vi "Add Step at Index.vi"(8 "error in (no error)":errorcluster, 9 "Step":refnum<class "Step.lvclass">, 10 "Index":i32, 11 "SequenceViewPanel in":refnum<class "SequenceViewPanel.lvclass">) -> (0 "error out":errorcluster, 1 "Step Group":T1, 2 "Parent Tag":string, 3 "SequenceViewPanel out":refnum<class "SequenceViewPanel.lvclass">)   [LabVIEW 2020, in "TSnax UI.lvlib" / "SequenceViewPanel.lvclass"]
uses:
  SequenceViewPanel.lvclass
  TSnax/Step/Step.lvclass
  TSnax/Step Group.ctl
  SequenceViewPanel.lvclass/SequenceViewPanel.ctl
  a9e04c75-c84a-4490-97d8-3532c9a77d1f.vi
  <vilib>/Comparison/Equal/Equal Functor/Equal Functor.lvclass
  TSnax/TSnax.lvlib
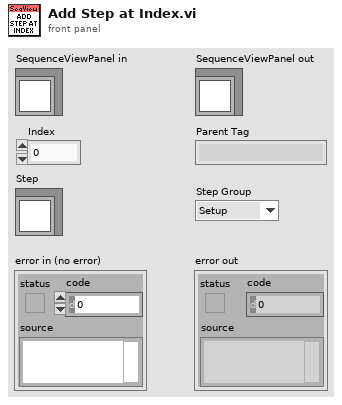
[diagram p1: front panel]
types:
  T1 = typedef "TSnax.lvlib/Step Group.ctl" = enum16{"Setup", "Main", "Cleanup"}
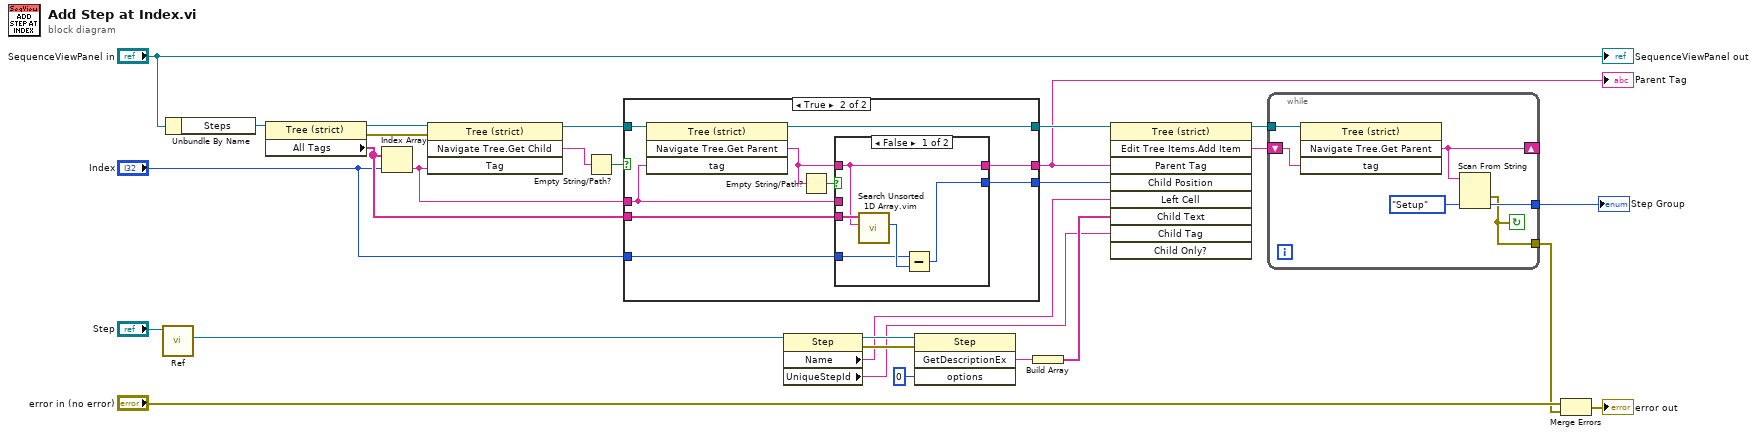
[diagram p0: block diagram]
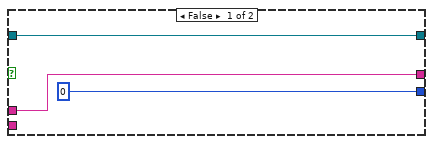
[diagram p2: hidden frame]
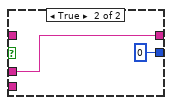
[diagram p3: hidden frame]
diagram:
  n1 = call "Ref.vi"("Step in"="Step") -> ("Step"=w7:refnum<k7>)  [unwired: 8 in, 2 out]
  n2 = Unbundle By Name("SequenceViewPanel in") -> ("Steps"=w26:refnum<vi>)
  n3 = property class="Tree (strict)"(reference=w26) -> (reference out=w25:refnum<vi>, error out=w10:errorcluster, "All Tags"=w20:string[])  [unwired: 1 in]
  n4 = Index Array(array=w20, index="Index") -> (element=w21:string)
  n5 = invoke class="Tree (strict)" method="Navigate Tree.Get Child"(reference=w25, error in=w10, "Tag"=w21) -> (reference out=w22:refnum<vi>, "Navigate Tree:Get Child"=w24:string)  [unwired: 1 in, 2 out]
  n6 = Empty String/Path?(string/path=w24) -> (empty?=w23:bool)
  n7 = case shown="True" w23 {
    tunnel: w22 -> [w29 w40]
    tunnel: w21 -> [w31 w33]
    tunnel: w20 -> [_ w39]
    tunnel: [w31 w35] -> w5
    tunnel: [0 w38] -> w19
    tunnel: [w29 w37] -> w18
    tunnel: "Index" -> [_ w32]
    frame False {
    }
    frame True {
      n8 = invoke class="Tree (strict)" method="Navigate Tree.Get Parent"(reference=w40, "tag"=w33) -> (reference out=w37:refnum<vi>, "Navigate Tree:Get Parent"=w36:string)  [unwired: 2 in, 2 out]
      n9 = Empty String/Path?(string/path=w36) -> (empty?=w34:bool)
      n10 = case shown="False" w34 {
        tunnel: w39 -> [w45 _]
        tunnel: [w43 0] -> w38
        tunnel: w36 -> [w42 _]
        tunnel: [w42 w47] -> w35
        tunnel: w33 -> [_ w47]
        tunnel: w32 -> [w41 _]
        frame False {
          n11 = call "Search Unsorted 1D Array.vim"("element"=w42, "unsorted 1D array"=w45) -> ("index of element"=w44:i32)  [unwired: 9 in]
          n12 = Subtract(x=w41, y=w44) -> (x-y=w43:i32)
        }
        frame True {
        }
      }
    }
  }
  "Parent Tag" <- w5
  n13 = property class="Step"(reference=w7) -> (reference out=w16:refnum<k7>, error out=w28:errorcluster, "Name"=w11:string, "UniqueStepId"=w12:string)  [unwired: 1 in]
  n14 = invoke class="Step" method="GetDescriptionEx"(reference=w16, error in=w28, "options"=0) -> ("GetDescriptionEx"=w14:string)  [unwired: 1 in, 3 out]
  n15 = Build Array(w14) -> (w13:string[])
  n16 = invoke class="Tree (strict)" method="Edit Tree Items.Add Item"(reference=w18, "Parent Tag"=w5, "Child Position"=w19, "Left Cell"=w11, "Child Text"=w13, "Child Tag"=w12) -> (reference out=w6:refnum<vi>, "Edit Tree Items:Add Item"=w4:string)  [unwired: 3 in, 7 out]
  n17 = while {
    tunnel: w6 -> [w53]
    shift-right: [w49] -> _
    shift-left: w4 -> [w52]
    tunnel: [w50] -> w3
    tunnel: [w48] -> w1
    stop <- w48 continue-if-true
    n18 = invoke class="Tree (strict)" method="Navigate Tree.Get Parent"(reference=w53, "tag"=w52) -> ("Navigate Tree:Get Parent"=w49:string)  [unwired: 2 in, 3 out]
    n19 = Scan From String(input string=w49, default 1=Step_Group."Setup" ("Step Group")) -> (error out=w48:errorcluster, output 1=w50:T1)  [unwired: 3 in, 2 out]
  }
  "Step Group" <- w3
  n20 = Merge Errors("error in (no error)", w1) -> (→"error out":errorcluster)
  "SequenceViewPanel out" <- "SequenceViewPanel in"
